vi "FileIO-Create Backup (rename).vi"(8 "error in (no error)":errorcluster, 10 "Delete tag":bool, 11 "Path":path) -> (0 "error out":errorcluster, 1 "backup created?":bool, 2 "Backup Path":path, 3 "Path (thru)":path)   [LabVIEW 2020]
uses:
  kernel32.dll
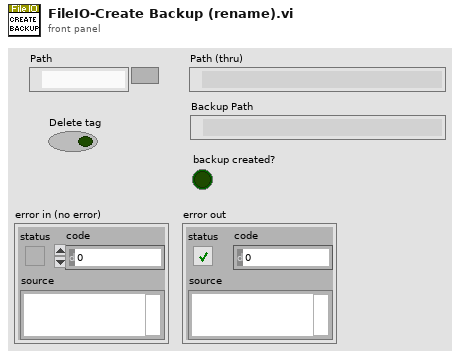
[diagram p1: front panel]
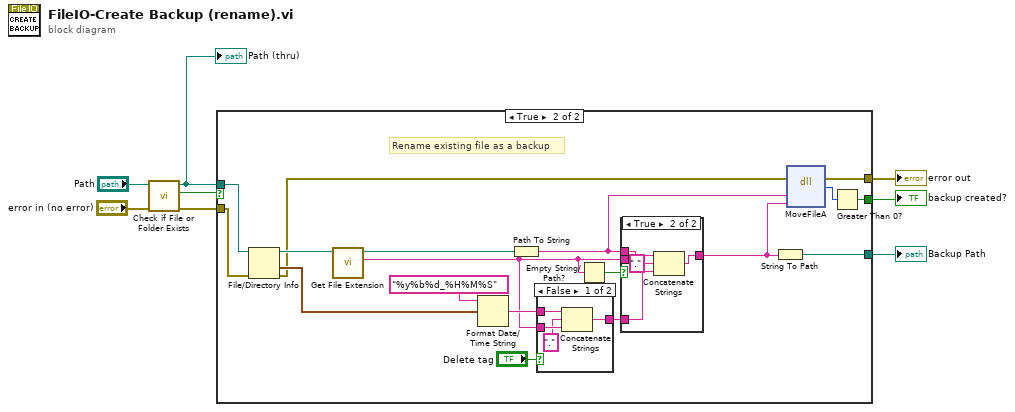
[diagram p0: block diagram]
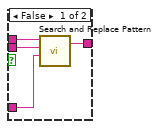
[diagram p3: hidden frame]
diagram:
  n1 = call <vilib>:"Check if File or Folder Exists.vi"("error in (no error)"="error in (no error)", "path"="Path") -> ("error out"=w5:errorcluster, "file or folder exists?"=w4:bool, "dup path"=w8:path)  [unwired: 7 in]
  "Path (thru)" <- w8
  n2 = case shown="True" w4 {
    tunnel: w8 -> [_ w23]
    tunnel: w5 -> [w9 w22]
    tunnel: [w9 w14] -> w6
    tunnel: [_ w21] -> w3
    tunnel: [_ w10] -> w1
    frame False {
    }
    frame True {
      # "Rename existing file as a backup"
      n3 = File/Directory Info(path=w23, error in=w22) -> (path out=w20:path, last mod=w24:timestamp, error out=w15:errorcluster)  [unwired: 4 out]
      n4 = call <vilib>:"Get File Extension.vi"("file"=w20) -> ("lowercase file extension"=w16:string, "dup file"=w19:path)  [unwired: 6 in, 3 out]
      n5 = Format Date/Time String(time format string (%c)="%y%b%d_%H%M%S", seconds (now)=w24) -> (date/time string=w27:string)  [unwired: 1 in]
      n6 = Path To String(path=w19) -> (string=w12:string)
      n7 = case shown="False" "Delete tag" {
        tunnel: w27 -> [w39 w40]
        tunnel: [w38 w40] -> w26
        tunnel: w16 -> [w37 _]
        frame False {
          n8 = Concatenate Strings(w39, "." ("string"), w37) -> (w38:string)
        }
        frame True {
        }
      }
      n9 = Empty String/Path?(string/path=w16) -> (empty?=w17:bool)
      n10 = case shown="True" w17 {
        tunnel: w12 -> [w31 w35]
        tunnel: w26 -> [w30 w33]
        tunnel: [w29 w34] -> w13
        tunnel: w16 -> [w28 _]
        frame False {
          n11 = call <vilib>:"Search and Replace Pattern.vi"("string"=w31, "regular expression (\"\")"=w28, "replace string (\"\")"=w30) -> ("result string"=w29:string)  [unwired: 2 in, 1 out]
        }
        frame True {
          n12 = Concatenate Strings(w35, "." ("string"), w33) -> (w34:string)
        }
      }
      n13 = String To Path(string=w13) -> (path=w21:path)
      n14 = dll-call lib="kernel32.dll" fn="MoveFileA"(error in=w15, "arg1"=w12, "arg2"=w13) -> (error out=w14:errorcluster, "return type"=w11:i32)  [unwired: 4 in, 1 out]
      n15 = Greater Than 0?(x=w11) -> (x > 0?=w10:bool)
    }
  }
  "error out" <- w6
  "Backup Path" <- w3
  "backup created?" <- w1
